vi "MainTriggerer.vi"(6 "Value to pass":enum16{"Trigger", "True", "False"}(ring), 8 "error in (no error)":errorcluster, 10 "Control Name":string="Get Stage Position", 11 "Microscope in":refnum<class "Microscope.lvclass">) -> (0 "error out":errorcluster, 2 "VI out":refnum<vi>, 3 "Microscope out":refnum<class "Microscope.lvclass">)   [LabVIEW 2012, in "Microscope.lvclass"]
uses:
  classes/Microscope.lvclass
panel:
  in  "name or relative path":string="Microscope.vi"
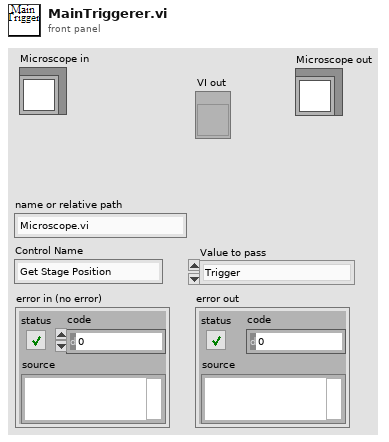
[diagram p1: front panel]
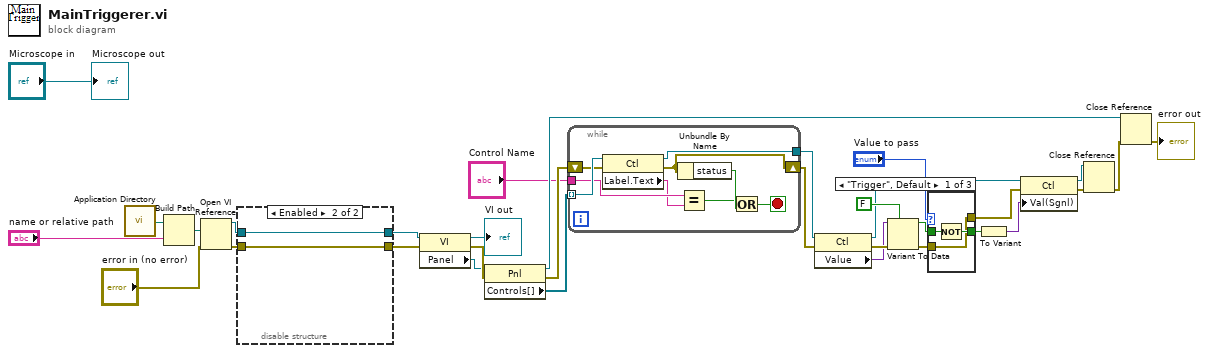
[diagram p0: block diagram]
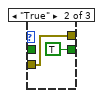
[diagram p2: hidden frame]
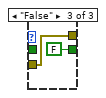
[diagram p3: hidden frame]
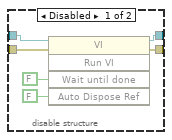
[diagram p4: hidden frame]
diagram:
  n1 = call <vilib>:"Application Directory.vi"() -> ("Application Directory"=w12:path)
  n2 = Build Path(base path=w12, name or relative path="name or relative path") -> (appended path=w11:path)
  n3 = Open VI Reference(vi path=w11, error in (no error)="error in (no error)") -> (vi reference=w10:refnum<vi>, error out=w9:errorcluster)  [unwired: 4 in]
  n4 = disable-structure shown="Enabled" {
    disable-tunnel: w10 -> [w36 w40]
    disable-tunnel: w9 -> [w35 w39]
    disable-tunnel: [w34 w40] -> w8
    disable-tunnel: [w33 w39] -> w7
    frame Disabled {
      n5 = invoke class="VI" method="Run VI"(reference=w36, error in=w35, "Wait until done"=FALSE ("Front Panel Window:Open"), "Auto Dispose Ref"=FALSE ("Auto Dispose Reference")) -> (reference out=w34:refnum<vi>, error out=w33:errorcluster)  [unwired: 1 in, 3 out]
    }
    frame Enabled {
    }
  }
  n6 = property class="VI"(reference=w8, error in=w7) -> (reference out=→"VI out":refnum<vi>, error out=w25:errorcluster, "Panel"=w14:refnum<vi>)
  n7 = property class="Pnl"(reference=w14, error in=w25) -> (reference out=w32:refnum<vi>, error out=w26:errorcluster, "Controls[]"=w15:refnum<vi>[])
  n8 = while {
    tunnel: w15 -> [w49] mode=indexing
    tunnel: "Control Name" -> [w48]
    tunnel: [w46] -> w16
    shift-right: [w44] -> w27
    shift-left: w26 -> [w45]
    stop <- w43 stop-if-true
    n9 = property class="Ctl"(reference=w49, error in=w45) -> (reference out=w46:refnum<vi>, error out=w44:errorcluster, "Label.Text"=w47:string)
    n10 = Unbundle By Name(w44) -> ("status"=w42:bool)
    n11 = Equal?(x=w48, y=w47) -> (x = y?=w41:bool)
    n12 = Or(x=w41, y=w42) -> (x .or. y?=w43:bool)
  }
  n13 = property class="Ctl"(reference=w16, error in=w27) -> (reference out=w17:refnum<vi>, error out=w23:errorcluster, "Value"=w19:variant)
  n14 = Variant To Data(error in=w23, type=FALSE ("Push Other VI's Button 2"), Variant=w19) -> (data=w22:bool, error out=w1:errorcluster)
  n15 = case shown="\"Trigger\", Default" "Value to pass" {
    tunnel: w22 -> [w52 _ _]
    tunnel: [w51 TRUE FALSE] -> w21
    tunnel: [w50 w53 w55] -> w2
    tunnel: w1 -> [w50 w53 w55]
    frame "Trigger", Default {
      n16 = Not(x=w52) -> (.not. x?=w51:bool)
    }
    frame "True" {
    }
    frame "False" {
    }
  }
  n17 = To Variant(anything=w21) -> (Variant=w18:variant)
  n18 = property class="Ctl"(reference=w17, error in=w2, "Val(Sgnl)"=w18) -> (reference out=w31:refnum<vi>, error out=w30:errorcluster)
  n19 = Close Reference(reference=w31, error in (no error)=w30) -> (error out=w28:errorcluster)
  n20 = Close Reference(reference=w32, error in (no error)=w28) -> (error out=→"error out":errorcluster)
  "Microscope out" <- "Microscope in"
